vi "grabber_mc_split_data.vi"(6 "channel":i8, 8 "error in (no error)":errorcluster, 10 "array in":u64[](array[numeric]), 11 "cluster in":T1={"reception"={"square size"=3, "offset"=0, "# squares out"=0, "left over"=[], "raps points length"=1, "raps left over"=[]}, "fft"={"reference"=[]}}) -> (0 "error out":errorcluster, 1 "MC array":u16[](array[numeric]), 2 "RAPS data":u64[](array[numeric]), 3 "cluster out":T1={"reception"={"square size"=3, "offset"=0, "# squares out"=0, "left over"=[], "raps points length"=7, "raps left over"=[]}, "fft"={"reference"=[]}}, 4 "empty MC array?":bool)   [LabVIEW 2010]
uses:
  motion_correction_cluster.ctl
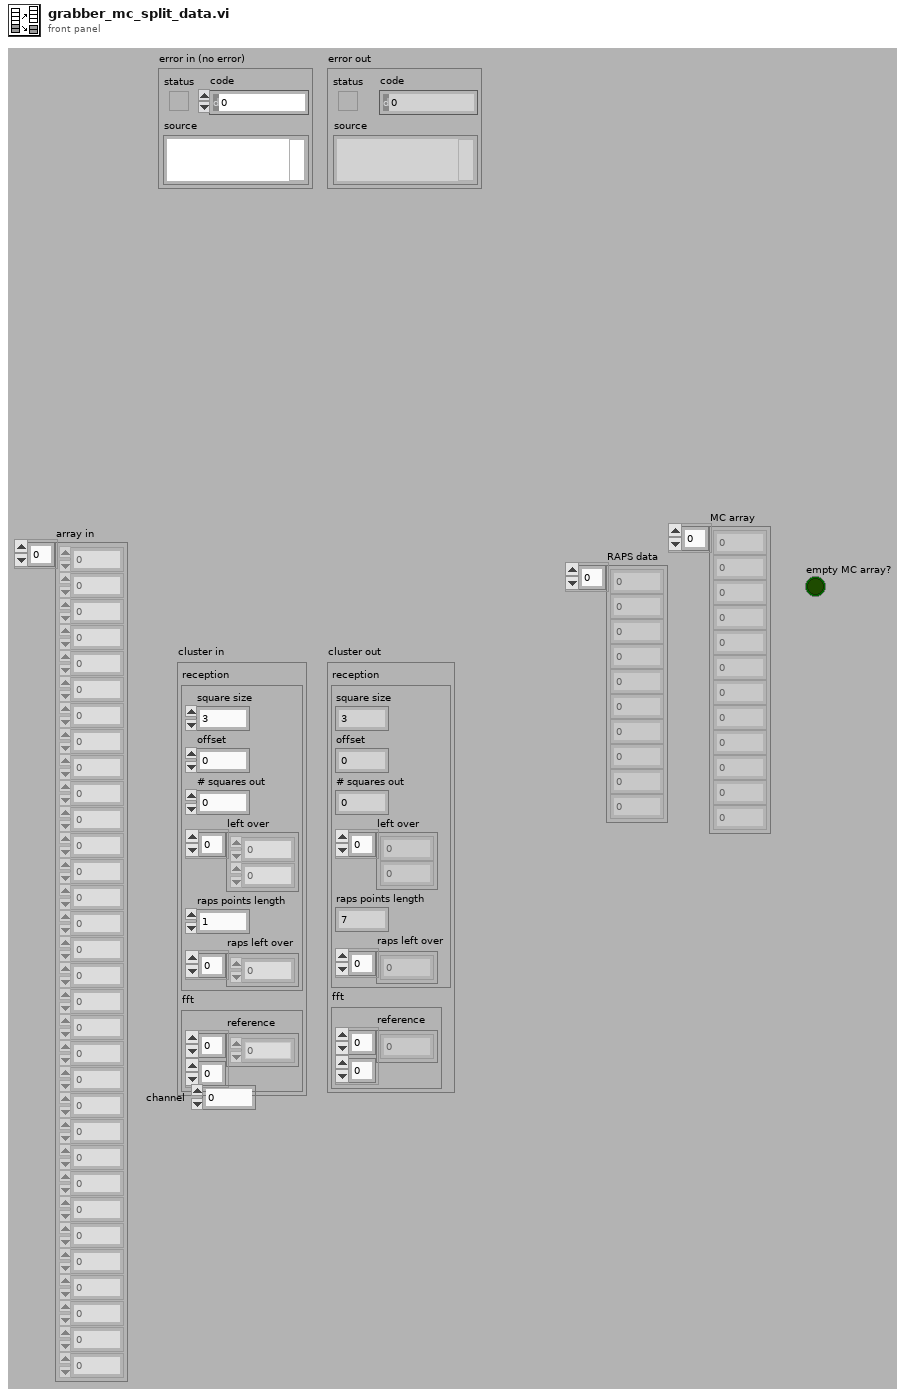
[diagram p1: front panel]
types:
  T1 = typedef "motion_correction_cluster.ctl" = cluster{"reception":cluster{"square size":i32, "offset":i32, "# squares out":i32, "left over":u16[], "raps points length":i32, "raps left over":u64[]}, "fft":cluster{"reference":dbl[][]}}
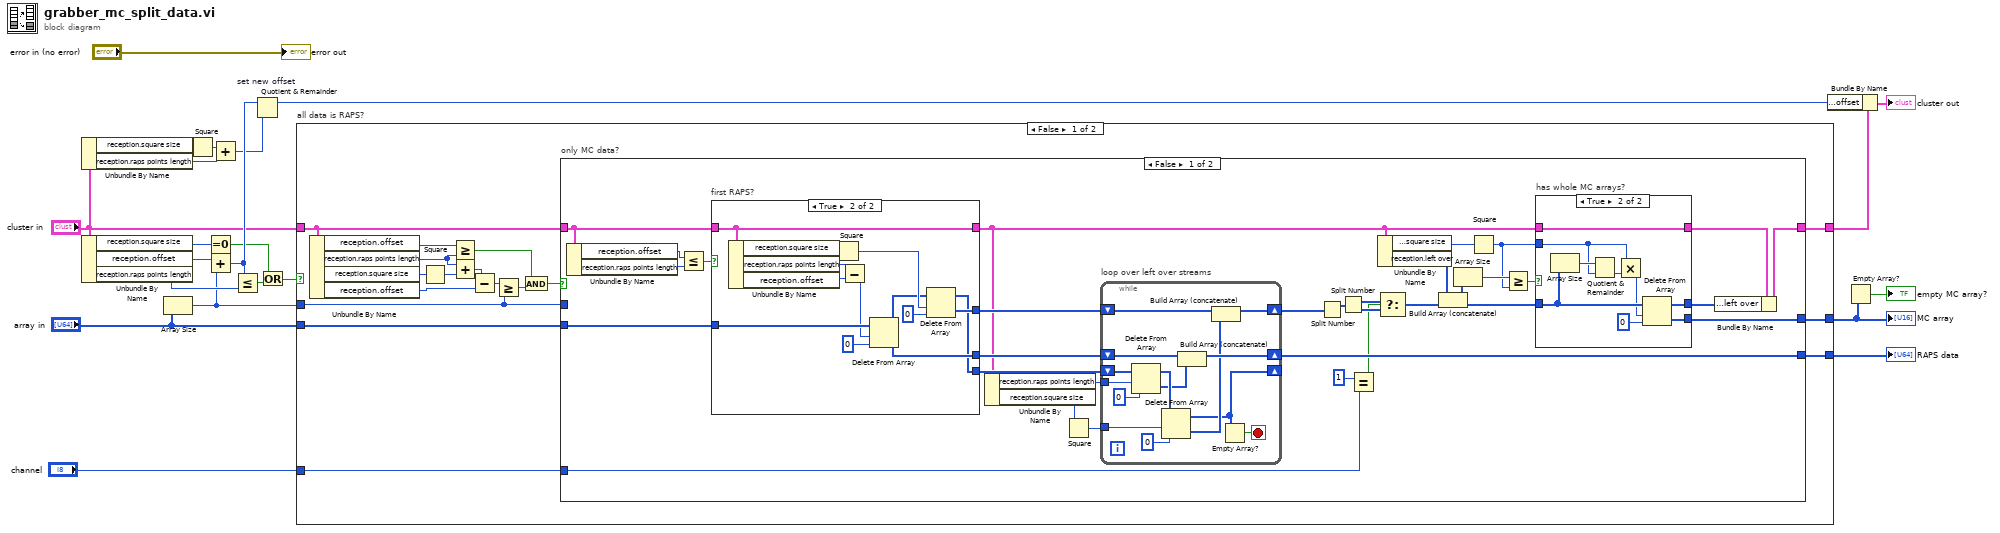
[diagram p0: block diagram]
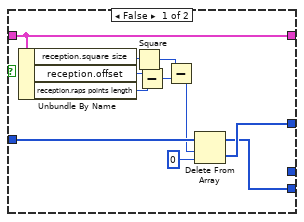
[diagram p3: hidden frame]
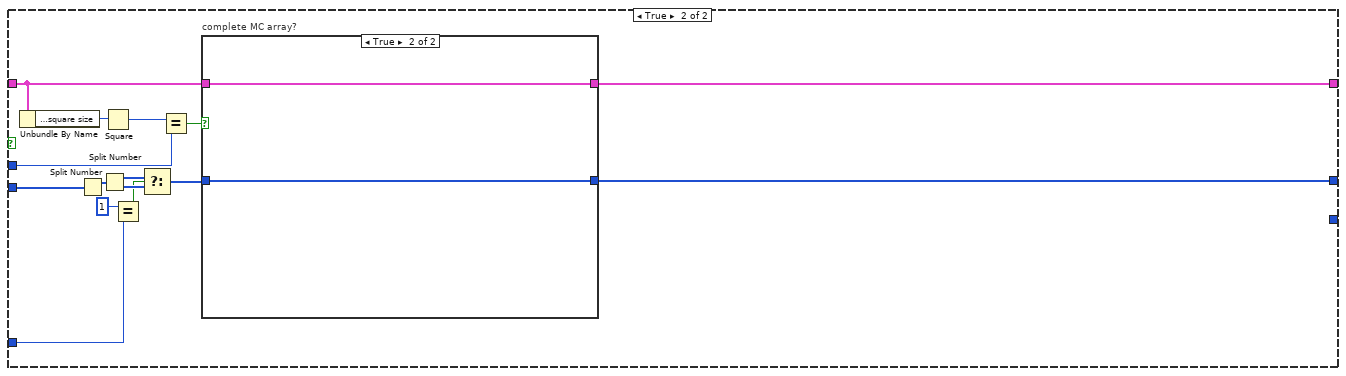
[diagram p4: hidden frame]
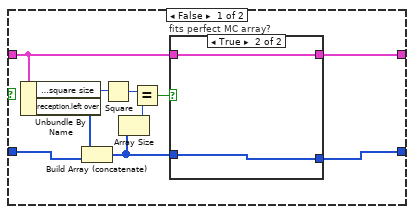
[diagram p5: hidden frame]
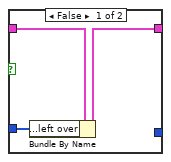
[diagram p6: hidden frame]
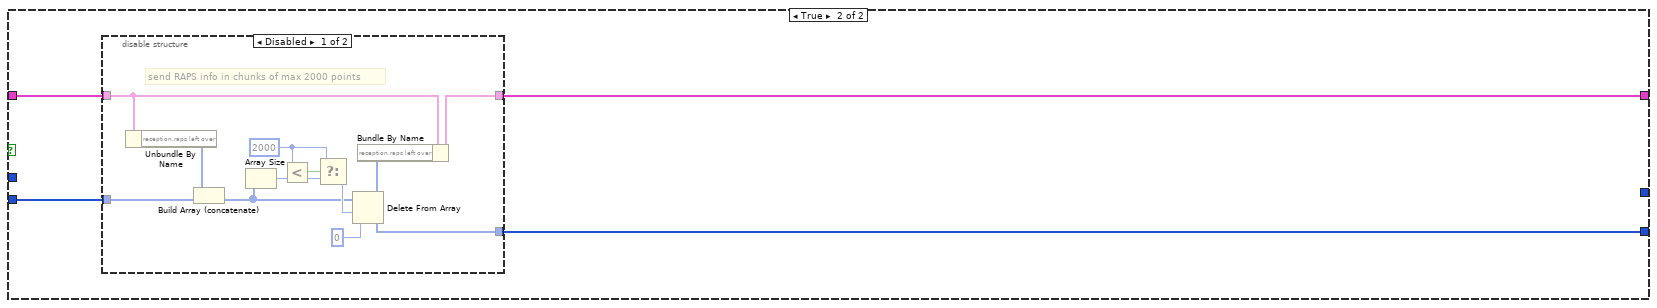
[diagram p7: hidden frame]
diagram:
  n1 = Unbundle By Name("cluster in") -> ("reception.square size"=w15:i32, "reception.raps points length"=w13:i32)
  n2 = Unbundle By Name("cluster in") -> ("reception.square size"=w2:i32, "reception.offset"=w20:i32, "reception.raps points length"=w19:i32)
  n3 = Array Size(array="array in") -> (size(s)=w18:i32)
  n4 = Square(x=w15) -> (x^2=w14:i32)
  n5 = Equal To 0?(x=w2) -> (x = 0?=w1:bool)
  n6 = Add(x=w20, y=w18) -> (x+y=w17:i32)
  n7 = Add(x=w14, y=w13) -> (x+y=w12:i32)
  n8 = Less Or Equal?(x=w17, y=w19) -> (x <= y?=w4:bool)
  n9 = Quotient & Remainder "set new offset"(x=w17, y=w12) -> (x-y*floor(x/y)=w11:i32)  [unwired: 1 out]
  n10 = Or(x=w1, y=w4) -> (x .or. y?=w3:bool)
  n11 = case "all data is RAPS?" shown="False" w3 {
    tunnel: "array in" -> [w34 w152]
    tunnel: [w26 w155] -> w8
    tunnel: "cluster in" -> [w27 w153]
    tunnel: w18 -> [w25 _]
    tunnel: [w35 _] -> w6
    tunnel: [w24 w154] -> w9
    tunnel: "channel" -> [w23 _]
    frame False {
      n12 = Unbundle By Name(w27) -> ("reception.offset"=w39:i32, "reception.raps points length"=w33:i32, "reception.square size"=w38:i32, "reception.offset"=w30:i32)
      n13 = Square(x=w38) -> (x^2=w32:i32)
      n14 = Greater Or Equal?(x=w39, y=w33) -> (x >= y?=w37:bool)
      n15 = Add(x=w33, y=w32) -> (x+y=w31:i32)
      n16 = Subtract(x=w31, y=w30) -> (x-y=w28:i32)
      n17 = Greater Or Equal?(x=w28, y=w25) -> (x >= y?=w29:bool)
      n18 = And(x=w37, y=w29) -> (x .and. y?=w36:bool)
      n19 = case "only MC data?" shown="False" w36 {
        tunnel: [w52 w130] -> w35
        tunnel: w34 -> [w67 w122]
        tunnel: w27 -> [w66 w129]
        tunnel: [w64 _] -> w26
        tunnel: w25 -> [_ w132]
        tunnel: [w48 w128] -> w24
        tunnel: w23 -> [w40 w120]
        frame False {
          n20 = Unbundle By Name(w66) -> ("reception.offset"=w70:i32, "reception.raps points length"=w69:i32)
          n21 = Less Or Equal?(x=w70, y=w69) -> (x <= y?=w68:bool)
          n22 = case "first RAPS?" shown="True" w68 {
            tunnel: w67 -> [w104 w117]
            tunnel: w66 -> [w96 w107]
            tunnel: [_ w115] -> w63
            tunnel: [w100 w108] -> w62
            tunnel: [w101 w110] -> w65
            tunnel: [w96 w107] -> w54
            frame False {
              n23 = Unbundle By Name(w96) -> ("reception.square size"=w106:i32, "reception.offset"=w99:i32, "reception.raps points length"=w98:i32)
              n24 = Square(x=w106) -> (x^2=w105:i32)
              n25 = Subtract(x=w99, y=w98) -> (x-y=w97:i32)
              n26 = Subtract(x=w105, y=w97) -> (x-y=w103:i32)
              n27 = Delete From Array(array=w104, length=w103, index=0) -> (deleted portion=w101:u64[], array with subset deleted=w100:u64[])
            }
            frame True {
              n28 = Unbundle By Name(w107) -> ("reception.square size"=w113:i32, "reception.raps points length"=w119:i32, "reception.offset"=w118:i32)
              n29 = Square(x=w113) -> (x^2=w112:i32)
              n30 = Subtract(x=w119, y=w118) -> (x-y=w116:i32)
              n31 = Delete From Array(array=w117, length=w116, index=0) -> (deleted portion=w115:u64[], array with subset deleted=w109:u64[])
              n32 = Delete From Array(array=w109, length=w112, index=0) -> (deleted portion=w110:u64[], array with subset deleted=w108:u64[])
            }
          }
          n33 = Unbundle By Name(w54) -> ("reception.raps points length"=w61:i32, "reception.square size"=w60:i32)
          n34 = Square(x=w60) -> (x^2=w59:i32)
          n35 = while "loop over left over streams" {
            tunnel: w61 -> [w89]
            tunnel: w59 -> [w87]
            shift-right: [w95] -> w42
            shift-left: w65 -> [w94]
            shift-right: [w93] -> w64
            shift-left: w63 -> [w92]
            shift-right: [w83] -> _
            shift-left: w62 -> [w91]
            stop <- w82 stop-if-true
            n36 = Delete From Array(array=w91, length=w89, index=0) -> (deleted portion=w84:u64[], array with subset deleted=w88:u64[])
            n37 = Delete From Array(array=w88, length=w87, index=0) -> (deleted portion=w85:u64[], array with subset deleted=w83:u64[])
            n38 = Build Array (concatenate)(w92, w84) -> (w93:u64[])
            n39 = Build Array (concatenate)(w94, w85) -> (w95:u64[])
            n40 = Empty Array?(array=w83) -> (empty?=w82:bool)
          }
          n41 = Split Number(x=w42) -> (hi(x)=w47:u32[])  [unwired: 1 out]
          n42 = Split Number(x=w47) -> (hi(x)=w43:u16[], lo(x)=w46:u16[])
          n43 = Equal?(x=i8 1 ("y"), y=w40) -> (x = y?=w44:bool)
          n44 = Unbundle By Name(w54) -> ("reception.square size"=w56:i32, "reception.left over"=w58:u16[])
          n45 = Select(t=w43, s=w44, f=w46) -> (s? t:f=w41:u16[])
          n46 = Build Array (concatenate)(w58, w41) -> (w53:u16[])
          n47 = Array Size(array=w53) -> (size(s)=w57:i32)
          n48 = Square(x=w56) -> (x^2=w51:i32)
          n49 = Greater Or Equal?(x=w57, y=w51) -> (x >= y?=w55:bool)
          n50 = case "has whole MC arrays?" shown="True" w55 {
            tunnel: [w71 w81] -> w49
            tunnel: w54 -> [w71 w81]
            tunnel: w53 -> [w72 w77]
            tunnel: [_ w74] -> w52
            tunnel: w51 -> [_ w79]
            tunnel: [w72 w73] -> w50
            frame False {
            }
            frame True {
              n51 = Array Size(array=w77) -> (size(s)=w80:i32)
              n52 = Quotient & Remainder(x=w80, y=w79) -> (floor(x/y)=w78:i32)  [unwired: 1 out]
              n53 = Multiply(x=w79, y=w78) -> (x*y=w75:i32)
              n54 = Delete From Array(array=w77, length=w75, index=0) -> (deleted portion=w74:u16[], array with subset deleted=w73:u16[])
            }
          }
          n55 = Bundle By Name(cluster=w49, "reception.left over"=w50) -> (w48:T1)
        }
        frame True {
          n56 = Unbundle By Name(w129) -> ("reception.square size"=w134:i32)
          n57 = Split Number(x=w122) -> (hi(x)=w127:u32[])  [unwired: 1 out]
          n58 = Split Number(x=w127) -> (hi(x)=w123:u16[], lo(x)=w126:u16[])
          n59 = Square(x=w134) -> (x^2=w133:i32)
          n60 = Equal?(x=i8 1 ("y"), y=w120) -> (x = y?=w124:bool)
          n61 = Select(t=w123, s=w124, f=w126) -> (s? t:f=w121:u16[])
          n62 = Equal?(x=w133, y=w132) -> (x = y?=w131:bool)
          n63 = case "complete MC array?" shown="True" w131 {
            tunnel: [w136 w151] -> w130
            tunnel: w121 -> [w135 w151]
            tunnel: w129 -> [w143 w150]
            tunnel: [w144 w150] -> w128
            frame False {
              n64 = Unbundle By Name(w143) -> ("reception.square size"=w141:i32, "reception.left over"=w142:u16[])
              n65 = Build Array (concatenate)(w142, w135) -> (w137:u16[])
              n66 = Square(x=w141) -> (x^2=w140:i32)
              n67 = Array Size(array=w137) -> (size(s)=w139:i32)
              n68 = Equal?(x=w140, y=w139) -> (x = y?=w138:bool)
              n69 = case "fits perfect MC array?" shown="True" w138 {
                tunnel: [w147 w148] -> w144
                tunnel: w143 -> [w146 w148]
                tunnel: w137 -> [w145 w149]
                tunnel: [_ w149] -> w136
                frame False {
                  n70 = Bundle By Name(cluster=w146, "reception.left over"=w145) -> (w147:T1)
                }
                frame True {
                }
              }
            }
            frame True {
            }
          }
        }
      }
    }
    frame True {
      n71 = disable-structure shown="Disabled" {
        disable-tunnel: [w163 w169] -> w155
        disable-tunnel: [w162 w168] -> w154
        disable-tunnel: w153 -> [w160 w168]
        disable-tunnel: w152 -> [w158 w169]
        frame Disabled {
          w165 = 2000 ("y")
          # "send RAPS info in chunks of max 2000 points"
          n72 = Unbundle By Name(w160) -> ("reception.raps left over"=w159:u64[])
          n73 = Build Array (concatenate)(w159, w158) -> (w157:u64[])
          n74 = Array Size(array=w157) -> (size(s)=w156:i32)
          n75 = Less?(x=w165, y=w156) -> (x < y?=w166:bool)
          n76 = Select(t=w165, s=w166, f=w156) -> (s? t:f=w164:i32)
          n77 = Delete From Array(array=w157, length=w164, index=0) -> (deleted portion=w163:u64[], array with subset deleted=w161:u64[])
          n78 = Bundle By Name(cluster=w160, "reception.raps left over"=w161) -> (w162:T1)
        }
        frame Enabled {
        }
      }
    }
  }
  "RAPS data" <- w8
  "MC array" <- w6
  n79 = Bundle By Name(cluster=w9, "reception.offset"=w11) -> (→"cluster out":T1)
  n80 = Empty Array?(array=w6) -> (empty?=→"empty MC array?":bool)
  "error out" <- "error in (no error)"
